vi "MakeFullPath.vi"(8 "エラー入力（エラーなし）":errorcluster, 11 "パス入力":path) -> (0 "エラー出力":errorcluster, 3 "パス出力":path)   [LabVIEW 2015]
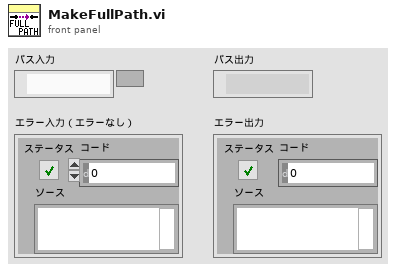
[diagram p1: front panel]
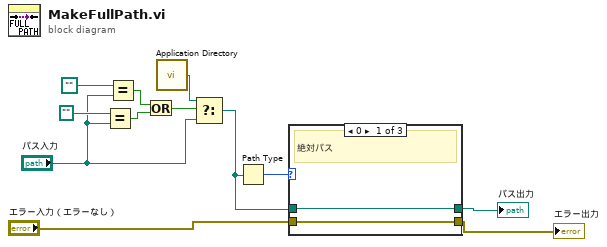
[diagram p0: block diagram]
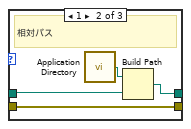
[diagram p2: hidden frame]
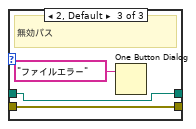
[diagram p3: hidden frame]
diagram:
  n1 = Equal?(x=path "", y="パス入力") -> (x = y?=w6:bool)
  n2 = Equal?(x=path "", y="パス入力") -> (x = y?=w5:bool)
  n3 = Or(x=w5, y=w6) -> (x .or. y?=w4:bool)
  n4 = call <vilib>:"Application Directory.vi"() -> ("Application Directory"=w3:path)
  n5 = Select(t=w3, s=w4, f="パス入力") -> (s? t:f=w1:path)
  n6 = Path Type(1:w1) -> (0:w9:i16)
  n7 = case shown="0" w9 {
    tunnel: w1 -> [w14 w17 w20]
    tunnel: [w14 w16 w20] -> w10
    tunnel: "エラー入力（エラーなし）" -> [w13 w15 w19]
    tunnel: [w13 w15 w19] -> w12
    frame 0 {
      # "絶対パス"
    }
    frame 1 {
      # "相対パス"
      n8 = call <vilib>:"Application Directory.vi"() -> ("Application Directory"=w18:path)
      n9 = Build Path(base path=w18, name or relative path=w17) -> (appended path=w16:path)
    }
    frame 2, Default {
      # "無効パス"
      n10 = One Button Dialog(message="ファイルエラー" ("メッセージ")) -> ()  [unwired: 1 in, 1 out]
    }
  }
  "エラー出力" <- w12
  "パス出力" <- w10
